vi "MeasurementType.Create.GlobalSettings.vi"(8 "error in (no error)":errorcluster, 9 "Name":string, 11 "Parent":T1 format="%.0x") -> (0 "error out":errorcluster, 2 "Child":T1 format="%.0x", 3 "Parent":T1 format="%.0x")   [LabVIEW 2015, in "Fuel Injector Analysis Addon System Explorer.lvlib"]
uses:
  <vilib>/NI Veristand/Custom Device API/Custom Device Item Ref.ctl
  Shared/Constants.vi
  <vilib>/NI Veristand/Custom Device Tools/Custom Device Utility Library/NI VeriStand - Search for Item by Name.vi
  Fuel Injector Analysis Addon System Explorer.lvlib
  <vilib>/NI Veristand/Custom Device Tools/Custom Device Utility Library/Custom Device Utility Library.lvlib
  <vilib>/NI VeriStand/Custom Device API/Custom Device API.lvlib
  Shared/Fuel Injector Analysis Addon Shared.lvlib
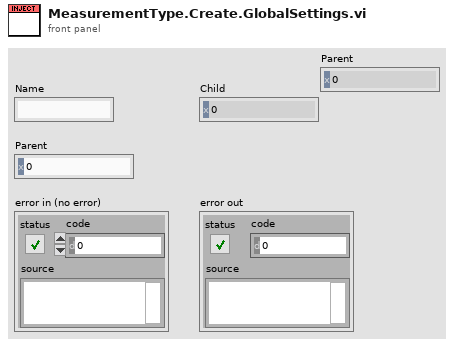
[diagram p1: front panel]
types:
  T1 = typedef "Custom Device API.lvlib/Custom Device Item Ref.ctl" = u64
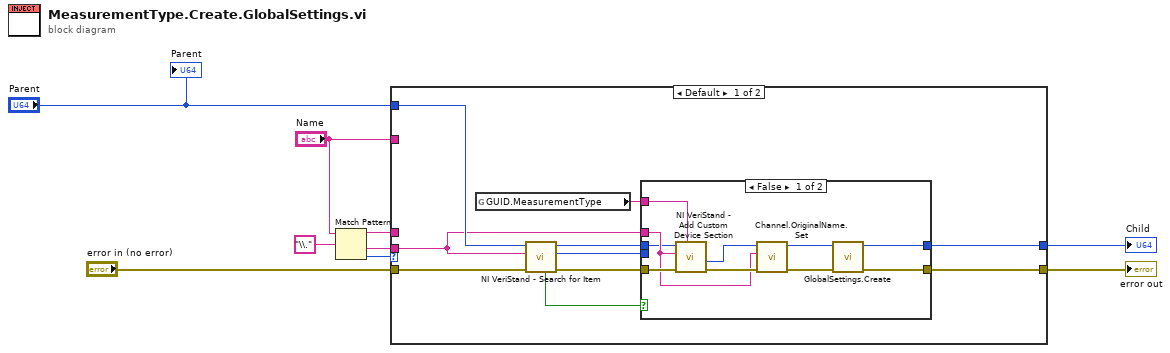
[diagram p0: block diagram]
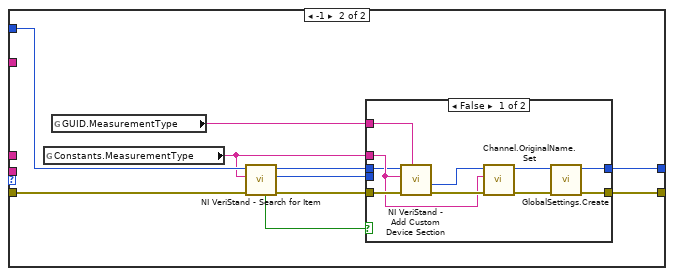
[diagram p3: hidden frame]
diagram:
  n1 = Match Pattern(string="Name", regular expression="\\.") -> (before substring=w4:string, after substring=w9:string, offset past match=w2:i32)  [unwired: 1 in, 1 out]
  n2 = case shown="Default" w2 {
    tunnel: "error in (no error)" -> [w19 w38]
    tunnel: w4 -> [_ _]
    tunnel: "Parent" -> [w18 w35]
    tunnel: [w14 w37] -> w5
    tunnel: [w13 w36] -> w7
    tunnel: "Name" -> [_ _]
    tunnel: w9 -> [w10 _]
    frame Default {
      n3 = global read "Constants.vi" "GUID.MeasurementType"() -> (w12:string)
      n4 = call-poly <vilib>:"NI VeriStand - Search for Item.vi"("error in"=w19, "Item Name"=w10, "Section Ref in"=w18) -> ("error out"=w17:errorcluster, "Item Ref"=w16:T1, "Section Ref out"=w11:T1, "Found"=w15:bool)  [unwired: 5 in]
      n5 = case shown="False" w15 {
        tunnel: w17 -> [w29 w31]
        tunnel: w16 -> [_ w30]
        tunnel: [w21 w31] -> w14
        tunnel: [w22 w30] -> w13
        tunnel: w10 -> [w25 _]
        tunnel: w12 -> [w28 _]
        tunnel: w11 -> [w20 _]
        frame False {
          n6 = call <vilib>:"NI VeriStand - Add Custom Device Section.vi"("GUID (Default Section)"=w28, "error in (no error)"=w29, "Section Name"=w25, "Parent Ref in"=w20) -> ("error out"=w27:errorcluster, "Section Ptr"=w26:T1)  [unwired: 4 in, 2 out]
          n7 = call "Channel.OriginalName.Set.vi"("error in (no error)"=w27, "Constants.Channel Name"=w25, "Ref"=w26) -> ("error out"=w24:errorcluster, "Ref out"=w23:T1)  [unwired: 7 in]
          n8 = call "GlobalSettings.Create.vi"("error in (no error)"=w24, "Device Item Ref in"=w23) -> ("error out"=w21:errorcluster, "Parent Ref out"=w22:T1)  [unwired: 8 in]
        }
        frame True {
        }
      }
    }
    frame -1 {
      n9 = global read "Constants.vi" "Constants.MeasurementType"() -> (w33:string)
      n10 = global read "Constants.vi" "GUID.MeasurementType"() -> (w34:string)
      n11 = call-poly <vilib>:"NI VeriStand - Search for Item.vi"("error in"=w38, "Item Name"=w33, "Section Ref in"=w35) -> ("error out"=w41:errorcluster, "Item Ref"=w40:T1, "Section Ref out"=w32:T1, "Found"=w39:bool)  [unwired: 5 in]
      n12 = case shown="False" w39 {
        tunnel: w41 -> [w51 w53]
        tunnel: w40 -> [_ w52]
        tunnel: [w43 w53] -> w37
        tunnel: [w44 w52] -> w36
        tunnel: w33 -> [w47 _]
        tunnel: w34 -> [w50 _]
        tunnel: w32 -> [w42 _]
        frame False {
          n13 = call <vilib>:"NI VeriStand - Add Custom Device Section.vi"("GUID (Default Section)"=w50, "error in (no error)"=w51, "Section Name"=w47, "Parent Ref in"=w42) -> ("error out"=w48:errorcluster, "Section Ptr"=w49:T1)  [unwired: 4 in, 2 out]
          n14 = call "Channel.OriginalName.Set.vi"("error in (no error)"=w48, "Constants.Channel Name"=w47, "Ref"=w49) -> ("error out"=w46:errorcluster, "Ref out"=w45:T1)  [unwired: 7 in]
          n15 = call "GlobalSettings.Create.vi"("error in (no error)"=w46, "Device Item Ref in"=w45) -> ("error out"=w43:errorcluster, "Parent Ref out"=w44:T1)  [unwired: 8 in]
        }
        frame True {
        }
      }
    }
  }
  "Child" <- w7
  "error out" <- w5
  "Parent" <- "Parent"
